vi "CheckCore.vi"(8 "error in (no error)":errorcluster, 9 "# of Refs":i32, 10 "References":refnum<vi>[](array[refnum]), 11 "Property in":refnum<class "Property.lvclass">) -> (0 "error out":errorcluster, 1 "Reject?":bool, 2 "dup References":refnum<vi>[](array[refnum]), 3 "Property out":refnum<class "Property.lvclass">)   [LabVIEW 2014, in "BuildSecurity.lvlib" / "Property.lvclass"]
doc: "Determines if any blacklisted property node exists in the VI."
uses:
  Property.lvclass
  Blacklist.lvclass/Blacklist.ctl
  ReadItems.vi
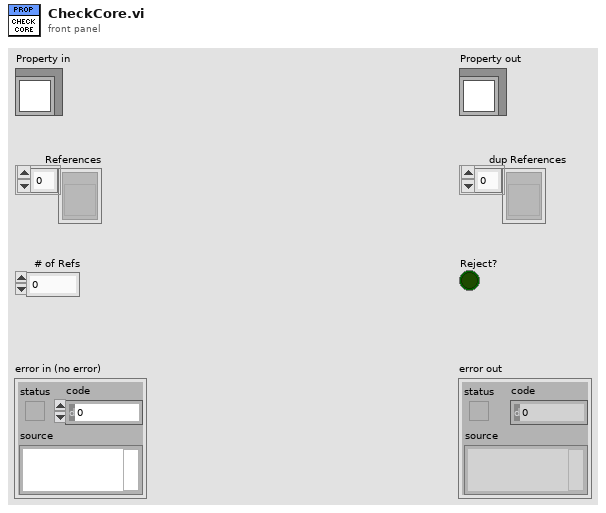
[diagram p1: front panel]
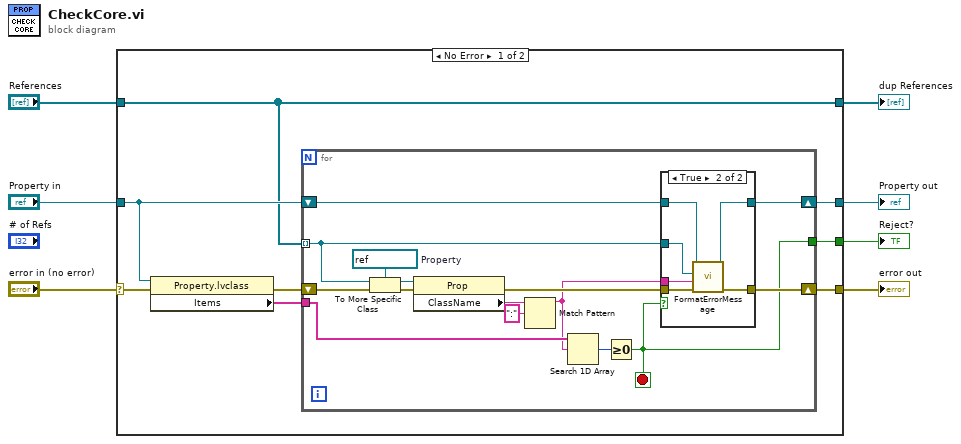
[diagram p0: block diagram]
diagram:
  n1 = case shown="No Error" "error in (no error)" {
    selector: "error in (no error)" -> [w15 w39]
    tunnel: "Property in" -> [w12 w41]
    tunnel: "References" -> [w11 w40]
    tunnel: [w11 w40] -> w2
    tunnel: [w10 _] -> w4
    tunnel: [w9 w39] -> w3
    tunnel: [w8 w41] -> w1
    frame No Error {
      n2 = property class="Property.lvclass"(reference=w12, error in=w15) -> (error out=w14:errorcluster, "Items"=w13:string[])  [unwired: 1 out]
      n3 = for {
        shift-right: [w17] -> w9
        shift-left: w14 -> [w24]
        tunnel: w13 -> [w23]
        shift-right: [w18] -> w8
        shift-left: w12 -> [w22]
        tunnel: w11 -> [w19] mode=indexing
        tunnel: [w16] -> w10
        stop <- w16 stop-if-true
        w30 = refnum<vi> refnum  # Property
        n4 = To More Specific Class(target class=w30, reference=w19, error in=w24) -> (specific class reference=w28:refnum<vi>, error out=w29:errorcluster)
        n5 = property class="Prop"(reference=w28, error in=w29) -> (error out=w21:errorcluster, "ClassName"=w26:string)  [unwired: 1 out]
        n6 = Match Pattern(string=w26, regular expression=":") -> (before substring=w20:string)  [unwired: 1 in, 3 out]
        n7 = Search 1D Array(1D array=w23, element=w20) -> (index of element=w27:i32)  [unwired: 1 in]
        n8 = Greater Or Equal To 0?(x=w27) -> (x >= 0?=w16:bool)
        n9 = case shown="True" w16 {
          tunnel: w22 -> [w32 w35]
          tunnel: w21 -> [w31 w38]
          tunnel: w20 -> [_ w37]
          tunnel: w19 -> [_ w36]
          tunnel: [w32 w34] -> w18
          tunnel: [w31 w33] -> w17
          frame False {
          }
          frame True {
            n10 = call-dynamic "FormatErrorMessage.vi"("error in (no error)"=w38, "Node qualifier"=w37, "GObj Refnum"=w36, "Blacklist in"=w35) -> ("error out"=w33:errorcluster, "Blacklist out"=w34:refnum<class "Property.lvclass">)  [unwired: 5 in, 1 out]
          }
        }
      }
    }
    frame Error {
    }
  }
  "error out" <- w3
  "Property out" <- w1
  "dup References" <- w2
  "Reject?" <- w4
